vi "Microcontroller_gopal.vi"() -> ()   [LabVIEW 2018]
uses:
  <vilib>/Utility/error.llb/DialogType.ctl
  <vilib>/MakerHub/LINX/Public/Peripherals/Digital/Digital Write 1 Chan.vi
  <vilib>/MakerHub/LINX/Public/Peripherals/Digital/Digital Write N Chans.vi
  <vilib>/MakerHub/LINX/Private/Local IO/LinxDigitalWrite.vi
  <vilib>/MakerHub/LINX/Public/Utilities/Check Channel.vi
  <vilib>/MakerHub/LINX/Public/Utilities/Open Serial.vi
  <vilib>/MakerHub/LINX/Private/Utilties/Generate Error.vi
  <vilib>/MakerHub/LINX/LMH-LINX.lvlib
panel:
  in  "Number of pulses":dbl
  in  "DO Channel":u8=9
  in  "Boolean":bool=TRUE
  in  "Direction":bool
  in  "DIrection Channel":u8=8
  in  "stop":bool
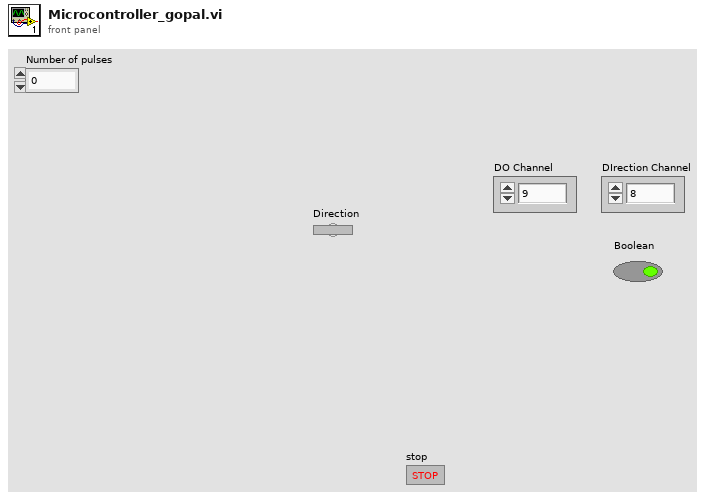
[diagram p1: front panel]
types:
  T1 = typedef "DialogType.ctl" = u16
  T2 = typedef "LMH-LINX.lvlib/LINX Ref.ctl" = cluster{"IO":T3, "Interface":T4, "LINX Device Config":T5}
  T3 = typedef "LMH-LINX.lvlib/Platform.ctl" = enum16{"Remote", "Local"}
  T4 = typedef "LMH-LINX.lvlib/Interface.ctl" = enum16{"Serial", "TCP"}
  T5 = typedef "LMH-LINX.lvlib/Device.lvlib/LINX Device Config.ctl" = cluster{"Interface":T4, "COM Port":refnum<visa-resource-name>, "TCP Configuration":T6, "Device Family":u8, "Device ID":u8, "Device Name":string, "TCP Ref":refnum<k5>, "Channels":T7}
  T6 = typedef "LMH-LINX.lvlib/Device.lvlib/TCP Config.ctl" = cluster{"IP Address":string, "Port":u16}
  T7 = typedef "LMH-LINX.lvlib/Channels.ctl" = cluster{"DI":u8[], "DO":u8[], "AI":u8[], "AO":u8[], "PWM":u8[], "QE":u8[], "UART":u8[], "I2C 2":u8[], "SPI":u8[], "CAN":u8[], "Servo":u8[], "AI Ref (V)":dbl, "AI Resolution (Bits)":u8, "AO Ref (V)":dbl, "AO Resolution (Bits)":u8}
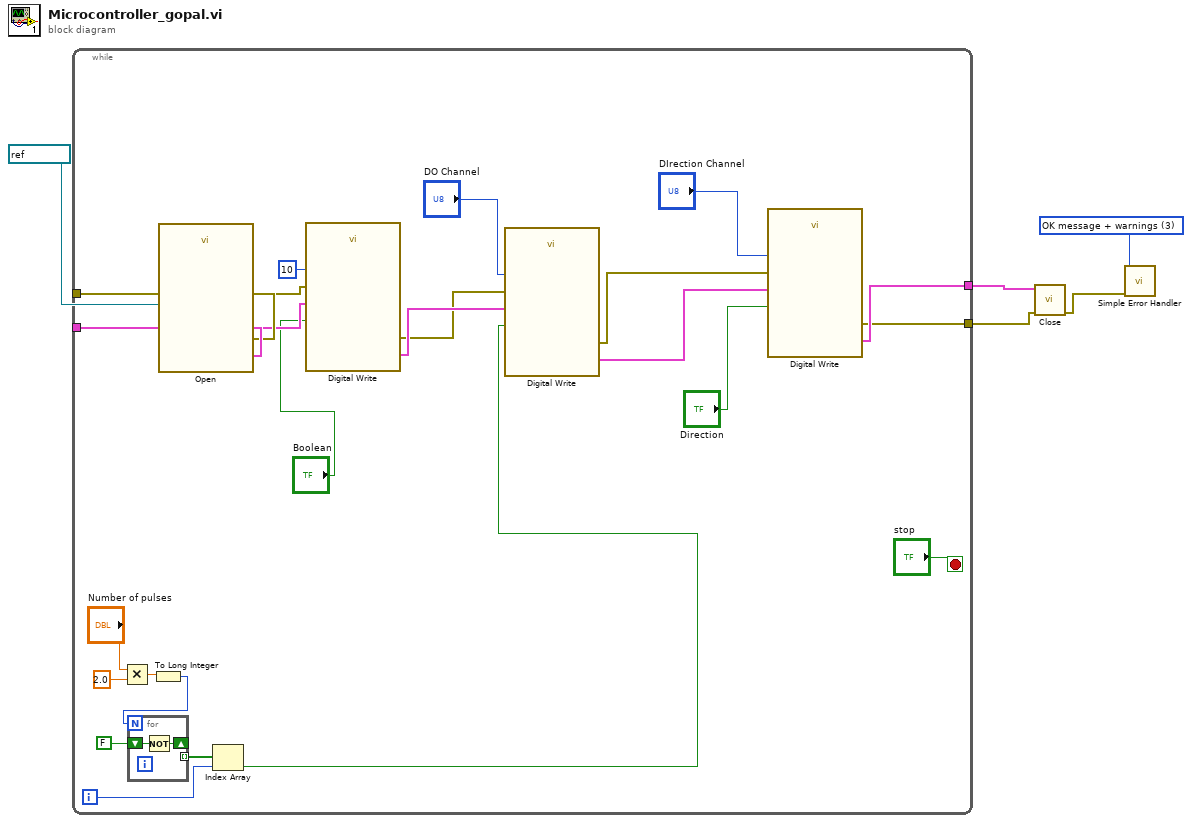
[diagram p0: block diagram]
diagram:
  w3 = T1 3 items=["no dialog", "OK message", "continue or stop message", "OK message + warnings", "continue/stop + warnings"] ("type of dialog (OK msg:1)")
  n1 = call-poly <vilib>:"Open.vi"("Serial Port"=refnum<visa-resource-name> "COM4") -> ("Error Out"=w5:errorcluster, "LINX Resource"=w6:T2)  [unwired: 8 in, 1 out]
  n2 = while {
    tunnel: w6 -> [w23]
    tunnel: w5 -> [w24]
    tunnel: [w26] -> w2
    tunnel: [w25] -> w1
    i -> [w12]
    stop <- "stop" stop-if-true
    n3 = Multiply(x="Number of pulses", y=2.0) -> (x*y=w9:dbl)
    n4 = To Long Integer(number=w9) -> (32bit integer=w8:i32)
    n5 = for {
      N: w8 -> [_]
      shift-right: [w30] -> _
      shift-left: FALSE -> [w31]
      tunnel: [w30] -> w15 mode=indexing
      n6 = Not(x=w31) -> (.not. x?=w30:bool)
    }
    n7 = Index Array(array=w15, index=w12) -> (element=w14:bool)
    n8 = call-poly <vilib>:"Digital Write.vi"("Error In"=w24, "Output Value"="Boolean", "DO Channel"=u8 10, "LINX Resource"=w23) -> ("Error Out"=w19:errorcluster, "LINX Resource"=w20:T2)  [unwired: 6 in]
    n9 = call-poly <vilib>:"Digital Write.vi"("Error In"=w19, "Output Value"=w14, "DO Channel"="DO Channel", "LINX Resource"=w20) -> ("Error Out"=w17:errorcluster, "LINX Resource"=w16:T2)  [unwired: 6 in]
    n10 = call-poly <vilib>:"Digital Write.vi"("Error In"=w17, "Output Value"="Direction", "DO Channel"="DIrection Channel", "LINX Resource"=w16) -> ("Error Out"=w25:errorcluster, "LINX Resource"=w26:T2)  [unwired: 6 in]
  }
  n11 = call <vilib>:"Close.vi"("Error In"=w1, "LINX Resource"=w2) -> ("Error Out"=w4:errorcluster)  [unwired: 9 in]
  n12 = call <vilib>:"Simple Error Handler.vi"("type of dialog (OK msg:1)"=w3, "error in (no error)"=w4) -> ()  [unwired: 3 in, 5 out]
